vi "find-vi-by-name.vi"(0 "Service Name (\"\":localhost)":string, 5 "Port(0:Ignored)":u16, 7 "Project Name (\"\": Main Application Instance)":string, 9 "VI Name":string, 11 "error in (no error)":errorcluster, 12 "Timeout ms (60000)":i32=60000) -> (4 "VI Reference":refnum<vi>, 15 "error out":errorcluster)   [LabVIEW 2016]
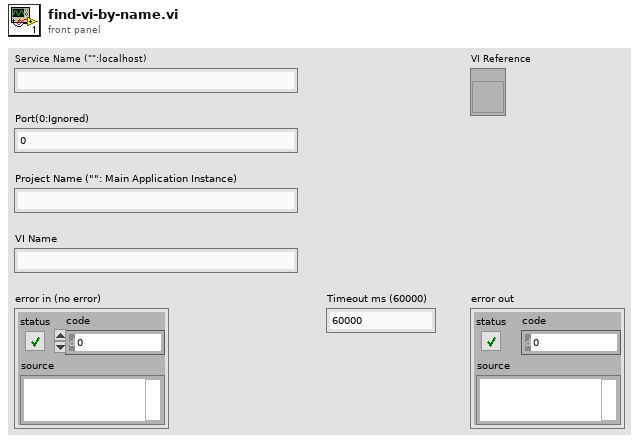
[diagram p1: front panel]
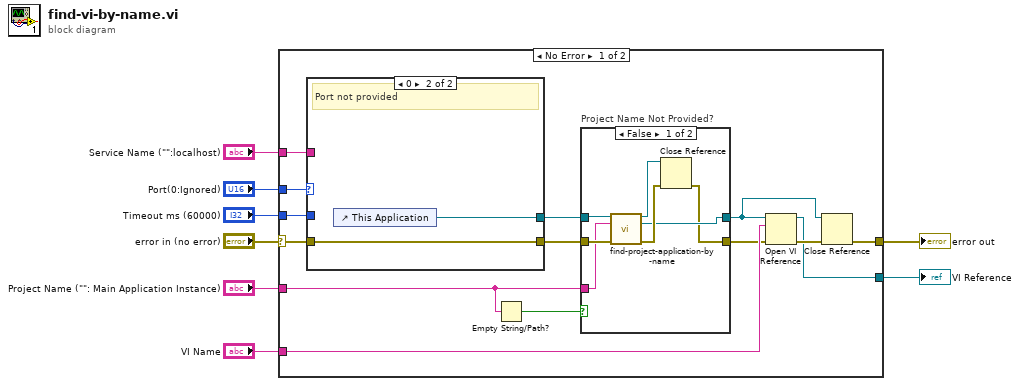
[diagram p0: block diagram]
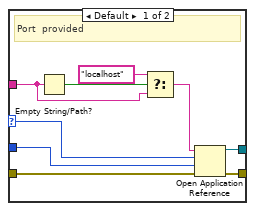
[diagram p3: hidden frame]
diagram:
  n1 = case shown="No Error" "error in (no error)" {
    selector: "error in (no error)" -> [w19 w43]
    tunnel: "Service Name (\"\":localhost)" -> [w22 _]
    tunnel: "Port(0:Ignored)" -> [w21 _]
    tunnel: "Timeout ms (60000)" -> [w20 _]
    tunnel: "VI Name" -> [w17 _]
    tunnel: [w16 _] -> w3
    tunnel: "Project Name (\"\": Main Application Instance)" -> [w15 _]
    tunnel: [w9 w43] -> w1
    frame No Error {
      n2 = case shown="0" w21 {
        selector: w21 -> [w40 _]
        tunnel: w20 -> [w39 _]
        tunnel: w19 -> [w38 w42]
        tunnel: [w33 w42] -> w13
        tunnel: w22 -> [w36 _]
        tunnel: [w32 w41] -> w10
        frame Default {
          # "Port  provided"
          n3 = Empty String/Path?(string/path=w36) -> (empty?=w37:bool)
          n4 = Select(t="localhost", s=w37, f=w36) -> (s? t:f=w34:string)
          n5 = Open Application Reference(8:w38, 9:w39, 10:w40, 11:w34) -> (0:w33:errorcluster, 3:w32:refnum<vi>)
        }
        frame 0 {
          # "Port not provided"
          n6 = control-ref of="This Application"() -> (w41:refnum<vi>)
        }
      }
      n7 = Empty String/Path?(string/path=w15) -> (empty?=w14:bool)
      n8 = case "Project Name Not Provided?" shown="False" w14 {
        tunnel: w15 -> [w27 _]
        tunnel: w13 -> [w29 w31]
        tunnel: [w24 w31] -> w12
        tunnel: [w25 w30] -> w11
        tunnel: w10 -> [w26 w30]
        frame False {
          n9 = call "find-project-application-by-name.vi"("Application Reference in"=w26, "Project Name"=w27, "error in (no error)"=w29) -> ("Application Reference out"=w23:refnum<vi>, "Project Application Ref"=w25:refnum<vi>, "error out"=w28:errorcluster)  [unwired: 10 in]
          n10 = Close Reference(reference=w23, error in (no error)=w28) -> (error out=w24:errorcluster)
        }
        frame True {
        }
      }
      n11 = Open VI Reference(application reference (local)=w11, vi path=w17, error in (no error)=w12) -> (vi reference=w16:refnum<vi>, error out=w18:errorcluster)  [unwired: 3 in]
      n12 = Close Reference(reference=w11, error in (no error)=w18) -> (error out=w9:errorcluster)
    }
    frame Error {
    }
  }
  "VI Reference" <- w3
  "error out" <- w1
